vi "Initialize PWM Output Channel Settings.vi"(11 "array size":i32=8) -> (3 "channel settings":T1[](array[typedef]))   [LabVIEW 2019, in "Module Test.lvclass"]
uses:
  Module Test Classes/Module Test.lvclass
  Scripting/Modules/Mode Classes/Controls/pwm channel settings.ctl
  Scripting/Modules/Channel Classes/PWM Output Channel/Frequency.ctl
  Scripting/Modules/Channel Classes/PWM Output Channel/PWM Output Channel.lvclass
  Scripting/Scan Engine Scripting.lvlib
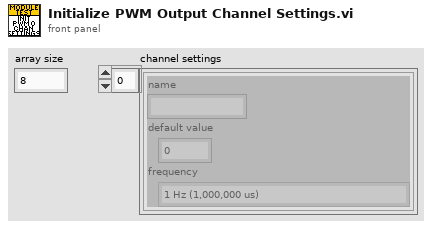
[diagram p1: front panel]
types:
  T1 = typedef "Scan Engine Scripting.lvlib/pwm channel settings.ctl" = cluster{"name":string, "default value":dbl, "frequency":T2}
  T2 = typedef "Scan Engine Scripting.lvlib/PWM Output Channel.lvclass/Frequency.ctl" = enum16{"1 Hz (1,000,000 us)", "50 Hz (20,000 us)", "250 Hz (4,000 us)", "500 Hz (2,000 us)", "1 kHz (1,000 us)", "5 kHz (200 us)", "10 kHz (100 us)", "20 kHz (50 us)"}
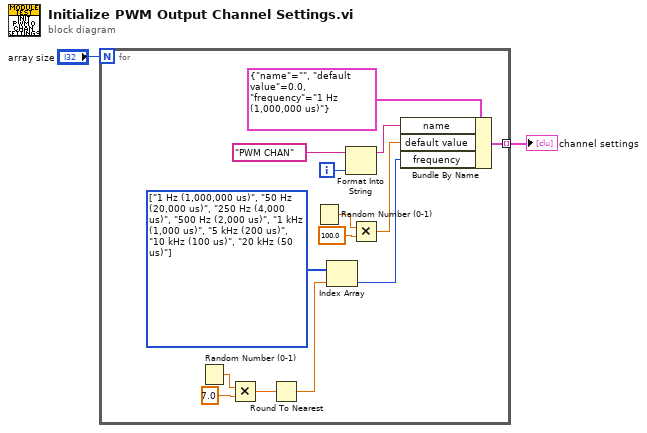
[diagram p0: block diagram]
diagram:
  n1 = for {
    N: "array size" -> [_]
    tunnel: [w15] -> w2 mode=indexing
    i -> [w5]
    w7 = T2[] [enum."1 Hz (1,000,000 us)", enum."50 Hz (20,000 us)", enum."250 Hz (4,000 us)", enum."500 Hz (2,000 us)", enum."1 kHz (1,000 us)", enum."5 kHz (200 us)", enum."10 kHz (100 us)", enum."20 kHz (50 us)"] items=["1 Hz (1,000,000 us)", "50 Hz (20,000 us)", "250 Hz (4,000 us)", "500 Hz (2,000 us)", "1 kHz (1,000 us)", "5 kHz (200 us)", "10 kHz (100 us)", "20 kHz (50 us)"]
    n2 = Random Number (0-1)() -> (number: 0 to 1=w10:dbl)
    n3 = Multiply(x=w10, y=7.0) -> (x*y=w9:dbl)
    n4 = Round To Nearest(number=w9) -> (nearest integer value=w8:dbl)
    n5 = Random Number (0-1)() -> (number: 0 to 1=w14:dbl)
    n6 = Index Array(array=w7, index=w8) -> (element=w6:T2)
    n7 = Format Into String(initial string="PWM CHAN", w5) -> (resulting string=w3:string)  [unwired: 2 in, 1 out]
    n8 = Multiply(x=w14, y=100.0) -> (x*y=w12:dbl)
    n9 = Bundle By Name(cluster=T1 {"name"="", "default value"=0.0, "frequency"=enum."1 Hz (1,000,000 us)"} ("channel settings"), "name"=w3, "default value"=w12, "frequency"=w6) -> (w15:T1)
  }
  "channel settings" <- w2
